vi "Reconnect Unit.vi"(8 "error in (no error)":errorcluster, 10 "Timeout (S)":dbl=60.0, 11 "ENET_BS120x in":refnum<class "ENET_BS120x.lvclass">) -> (0 "error out":errorcluster, 3 "ENET_BS120x out":refnum<class "ENET_BS120x.lvclass">)   [LabVIEW 2021, in "BS120x Driver.lvlib" / "ENET_BS120x.lvclass"]
uses:
  ENET_BS120x.lvclass
panel:
  out "Num Tries":i32
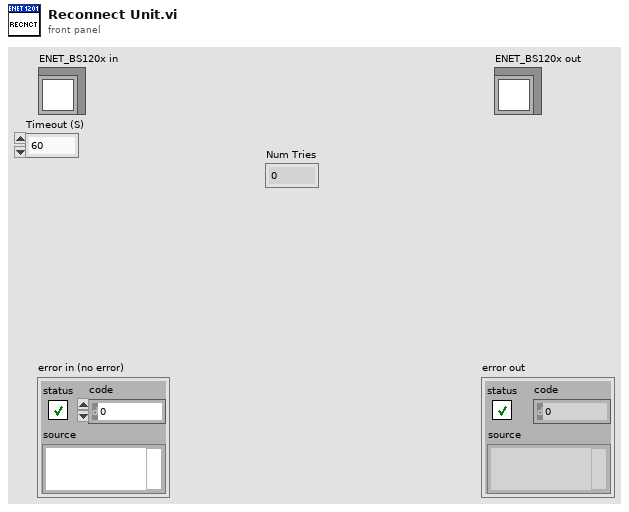
[diagram p1: front panel]
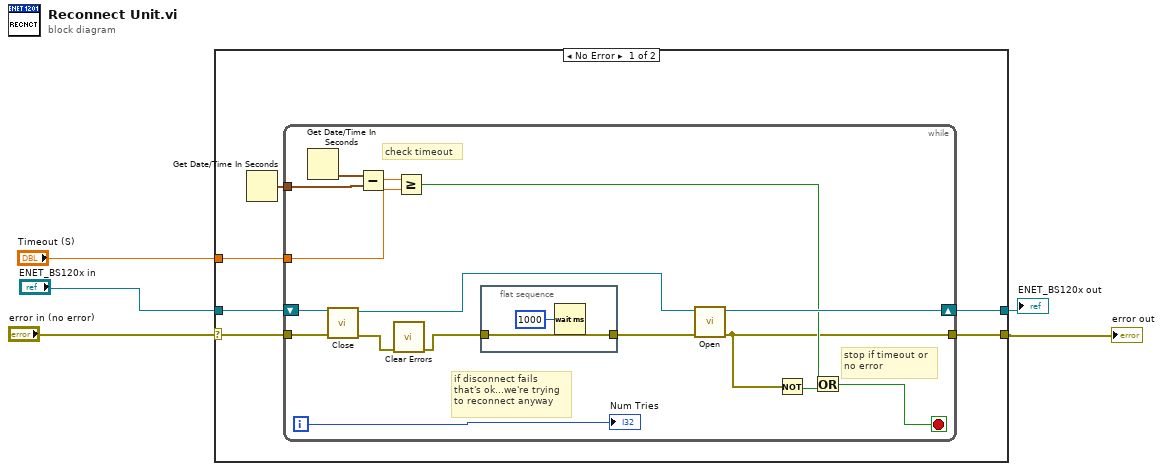
[diagram p0: block diagram]
diagram:
  n1 = case shown="No Error" "error in (no error)" {
    selector: "error in (no error)" -> [w8 w30]
    tunnel: [w11 w30] -> w4
    tunnel: [w10 w31] -> w2
    tunnel: "ENET_BS120x in" -> [w9 w31]
    tunnel: "Timeout (S)" -> [w7 _]
    frame No Error {
      n2 = Get Date/Time In Seconds() -> (seconds since 1Jan1904=w6:timestamp)
      n3 = while {
        tunnel: w7 -> [w16]
        shift-right: [w27] -> w10
        shift-left: w9 -> [w25]
        tunnel: w8 -> [w24]
        tunnel: [w13] -> w11
        tunnel: w6 -> [w19]
        i -> [w20]
        stop <- w12 stop-if-true
        # "stop if timeout or\nno error"
        # "check timeout"
        # "if disconnect fails\nthat's ok...we're trying\nto reconnect anyway"
        n4 = Get Date/Time In Seconds() -> (seconds since 1Jan1904=w18:timestamp)
        n5 = call-dynamic "Close.vi"("error in (no error)"=w24, "ENET in"=w25) -> ("error out"=w26:errorcluster, "ENET out"=w23:refnum<class "ENET_BS120x.lvclass">)  [unwired: 8 in]
        n6 = Subtract(x=w18, y=w19) -> (x-y=w17:dbl)
        n7 = call <vilib>:"Clear Errors.vi"("error in (no error)"=w26) -> ("error out"=w22:errorcluster)  [unwired: 5 in, 1 out]
        n8 = Greater Or Equal?(x=w17, y=w16) -> (x >= y?=w15:bool)
        n9 = flat-sequence {
          tunnel: [w29] -> w21
          tunnel: w22 -> [w29]
          frame #0 {
            n10 = Wait (ms)(milliseconds to wait=u32 1000) -> ()  [unwired: 1 out]
          }
        }
        n11 = call-dynamic "Open.vi"("error in (no error)"=w21, "ENET In"=w23) -> ("error out"=w13:errorcluster, "ENET out"=w27:refnum<class "ENET_BS120x.lvclass">)  [unwired: 8 in]
        n12 = Not(x=w13) -> (.not. x?=w14:bool)
        n13 = Or(x=w15, y=w14) -> (x .or. y?=w12:bool)
        "Num Tries" <- w20
      }
    }
    frame Error {
    }
  }
  "error out" <- w4
  "ENET_BS120x out" <- w2
